vi "Initialize.vi"(7 "fluidics line":string="Dev1/port2/line6", 8 "error in (no error)":errorcluster, 9 "Shutter Lines":string[](array[string]), 10 "Sync Line":string, 11 "Synchronization Device in":refnum<class "NI DAQ.lvclass">) -> (0 "error out":errorcluster, 3 "Synchronization Device out":refnum<class "NI DAQ.lvclass">)   [LabVIEW 2023, in "NI DAQ.lvlib" / "NI DAQ.lvclass"]
uses:
  NI DAQ.lvclass
  Resources/Type Defs/sync device settings.ctl
  NI DAQ.lvclass/NI DAQ.ctl
  <vilib>/DAQmx/create/channels.llb/DAQmx Create Channel (DO-Digital Output).vi
  <resource>/objmgr/daqmx.rc
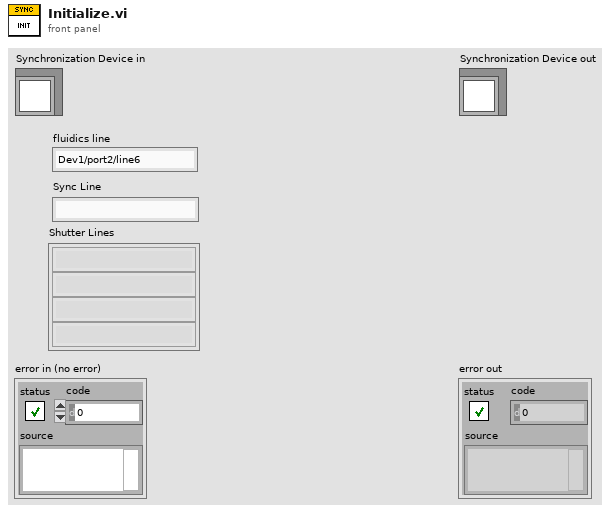
[diagram p1: front panel]
types:
  T1 = typedef "sync device settings.ctl" = cluster{"Interval (ms)":dbl, "ALEX":bool, "Shutter Enable":bool[], "Stream":bool, "Duty Cycle":dbl, "fluidics trigger frame":u16, "Frames to Skip":u32}
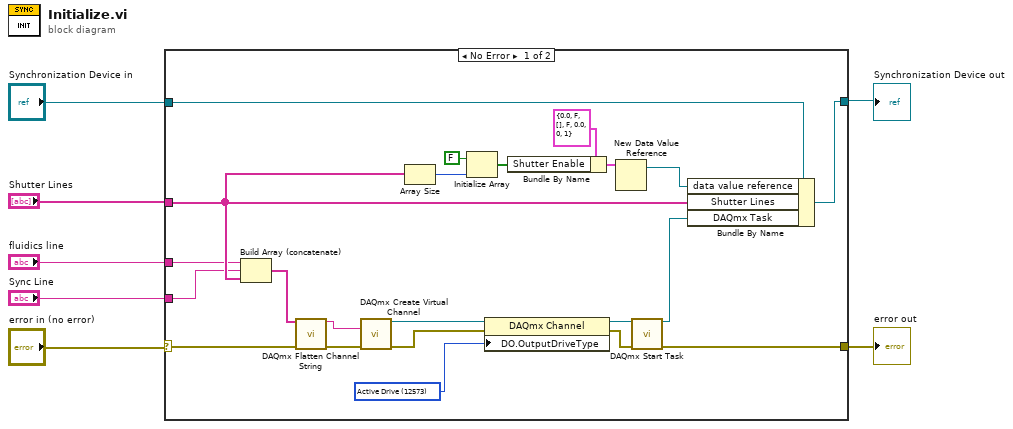
[diagram p0: block diagram]
diagram:
  n1 = case shown="No Error" "error in (no error)" {
    selector: "error in (no error)" -> [w17 w31]
    tunnel: [w18 w31] -> w6
    tunnel: [w28 w30] -> w4
    tunnel: "Synchronization Device in" -> [w29 w30]
    tunnel: "Sync Line" -> [w9 _]
    tunnel: "Shutter Lines" -> [w16 _]
    tunnel: "fluidics line" -> [w13 _]
    frame No Error {
      w19 = 12573 items=["Active Drive"=12573, "Open Collector"=12574] ("DO.OutputDriveType")
      n2 = Build Array (concatenate)(w13, w9, w16) -> (w22:string[])
      n3 = call <vilib>:"DAQmx Flatten Channel String.vi"("names in"=w22, "error in"=w17) -> ("names out"=w21:string, "error out"=w20:errorcluster)  [unwired: 12 in]
      n4 = call-poly <vilib>:"DAQmx Create Virtual Channel.vi"("lines"=w21, "error in"=w20) -> ("task out"=w26:refnum<k21>, "error out"=w24:errorcluster)  [unwired: 12 in]
      n5 = Array Size(array=w16) -> (size(s)=w12:i32)
      n6 = Initialize Array(FALSE, w12) -> (w15:bool[])
      n7 = property class="DAQmx Channel"(reference=w26, error in=w24, "DO.OutputDriveType"=w19) -> (reference out=w25:refnum<k21>, error out=w23:errorcluster)
      n8 = Bundle By Name(cluster=T1 {"Interval (ms)"=0.0, "ALEX"=FALSE, "Shutter Enable"=[], "Stream"=FALSE, "Duty Cycle"=0.0, "fluidics trigger frame"=0, "Frames to Skip"=1} ("input cluster"), "Shutter Enable"=w15) -> (w27:T1)
      n9 = New Data Value Reference(data value=w27) -> (data value reference=w14:refnum<data-value>)  [unwired: 1 in, 1 out]
      n10 = call <vilib>:"DAQmx Start Task.vi"("task/channels in"=w25, "error in"=w23) -> ("task out"=w10:refnum<k21>, "error out"=w18:errorcluster)  [unwired: 12 in]
      n11 = Bundle By Name(cluster=w29, "data value reference"=w14, "Shutter Lines"=w16, "DAQmx Task"=w10) -> (w28:refnum<class "NI DAQ.lvclass">)
    }
    frame Error {
    }
  }
  "error out" <- w6
  "Synchronization Device out" <- w4
